vi "Rename Help Files.vi"(8 "error in":errorcluster, 9 "CD name":string, 10 "relative path of Help files":path[](array[path]), 11 "custom device path":path) -> (0 "error out":errorcluster, 3 "custom device path out":path)   [LabVIEW 2020, in "Template Tool.lvlib"]
uses:
  Template Tool.lvlib
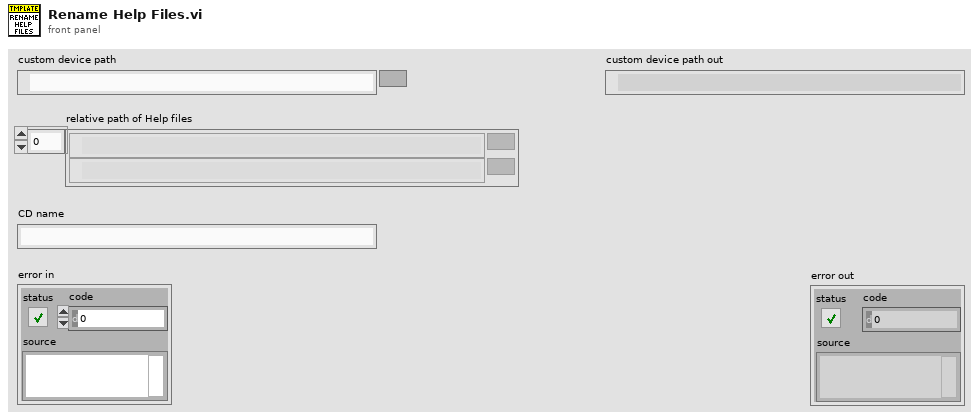
[diagram p1: front panel]
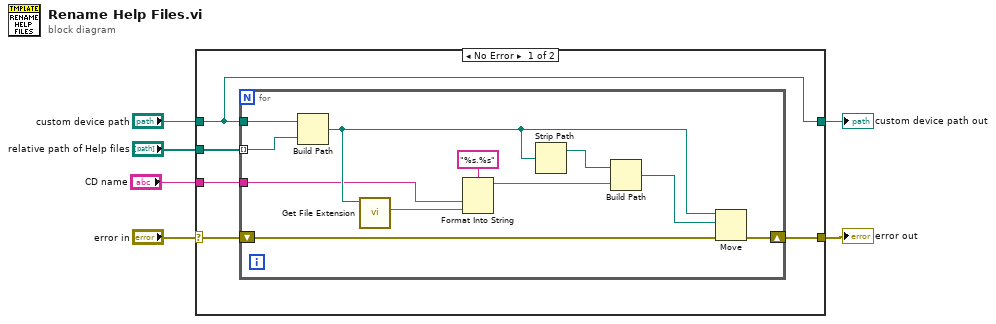
[diagram p0: block diagram]
diagram:
  n1 = case shown="No Error" "error in" {
    selector: "error in" -> [w11 w24]
    tunnel: "custom device path" -> [w9 w23]
    tunnel: [w10 w24] -> w5
    tunnel: [w9 w23] -> w4
    tunnel: "relative path of Help files" -> [w8 _]
    tunnel: "CD name" -> [w7 _]
    frame No Error {
      n2 = for {
        tunnel: w9 -> [w22]
        tunnel: w8 -> [w19] mode=indexing
        shift-right: [w20] -> w10
        shift-left: w11 -> [w21]
        tunnel: w7 -> [w12]
        n3 = Build Path(base path=w22, name or relative path=w19) -> (appended path=w16:path)
        n4 = call <vilib>:"Get File Extension.vi"("file"=w16) -> ("lowercase file extension"=w18:string)  [unwired: 6 in, 4 out]
        n5 = Format Into String(format string="%s.%s", w12, w18) -> (resulting string=w15:string)  [unwired: 2 in, 1 out]
        n6 = Strip Path(path=w16) -> (stripped path=w14:path)  [unwired: 1 out]
        n7 = Build Path(base path=w14, name or relative path=w15) -> (appended path=w13:path)
        n8 = Move(source path=w16, error in=w21, 10:w13) -> (error out=w20:errorcluster)  [unwired: 2 in, 2 out]
      }
    }
    frame Error {
    }
  }
  "error out" <- w5
  "custom device path out" <- w4
